vi "getAnonymousCredentials.vi"(11 "Connection.LocalQueue":refnum<class "Connection.LocalQueue.lvclass">) -> (1 "Anonymous password":string, 2 "Anonymous username":string)   [LabVIEW 2013, in "Connection.Queue_GOSPL.lvlib" / "Connection.LocalQueue.lvclass"]
uses:
  Connection.LocalQueue.lvclass
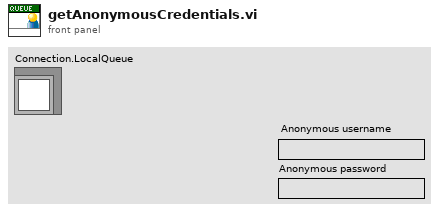
[diagram p1: front panel]
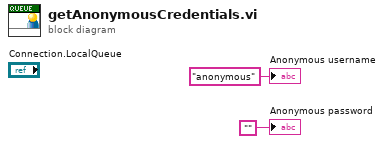
[diagram p0: block diagram]
diagram:
  "Anonymous username" <- "anonymous" ("Anonymous username")
  "Anonymous password" <- ""
